vi "NI VeriStand - Get Stimulus Profile Manager State.vi"(8 "error in (no error)":errorcluster, 11 "StimulusProfileManager in":T2) -> (0 "error out":errorcluster, 2 "State":T1, 3 "StimulusProfileManager out":T2)   [LabVIEW 2020, in "NI_VS Stimulus ExecutionAPI.lvlib"]
doc: "This VI interfaces with the legacy Stimulus Profile Editor workspace tool in NI VeriStand, and is included for compatibility only. National Instruments recommends you use the current Stimulus Profile VIs to create, observe, and control NI VeriStand stimulus profiles and real-time sequences.\n\nReturns the status of the stimulus profile manager, including whether it is stopped, starting, running, or stopping."
uses:
  <vilib>/NI VeriStand/Execution/Stimulus/NI_VS Stimulus ExecutionAPI.lvlib
  <vilib>/NI VeriStand/Execution/Stimulus/StimulusAPI.ctl
  NationalInstruments.VeriStand.ClientAPI
  <vilib>/NI VeriStand/Execution/Stimulus/StimulusState.ctl
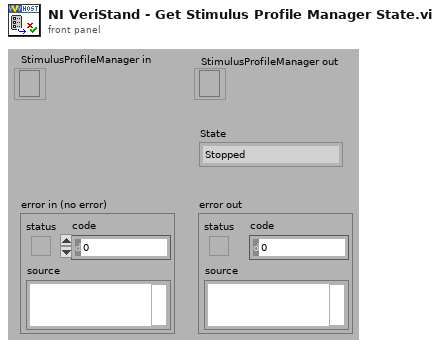
[diagram p1: front panel]
types:
  T1 = typedef "NI_VS Stimulus ExecutionAPI.lvlib/StimulusState.ctl" = enum16{"Stopped", "Starting", "Running", "Stopping"}
  T2 = typedef "NI_VS Stimulus ExecutionAPI.lvlib/StimulusAPI.ctl" = refnum<k24>
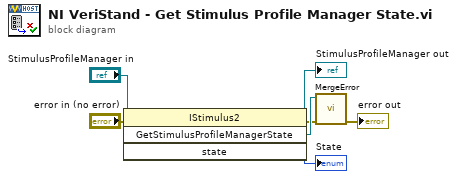
[diagram p0: block diagram]
diagram:
  n1 = invoke class="IStimulus2" method="GetStimulusProfileManagerState"(reference="StimulusProfileManager in", error in="error in (no error)") -> (reference out=→"StimulusProfileManager out":T2, error out=w3:errorcluster, "GetStimulusProfileManagerState"=w4:refnum<k24>, "state"=→"State":u8)  [unwired: 2 in]
  n2 = call <vilib>:"MergeError.vi"("error in (no error)"=w3, "Error"=w4) -> ("error out"=→"error out":errorcluster)  [unwired: 9 out]
